vi "Begin.vi"(8 "error in (no error)":errorcluster, 11 "Elevator Concrete in":refnum<class "Elevator Concrete.lvclass">) -> (0 "error out":errorcluster, 3 "Elevator Concrete out":refnum<class "Elevator Concrete.lvclass">)   [LabVIEW 2018, in "Elevator.lvlib" / "Elevator Concrete.lvclass"]
uses:
  Elevator Concrete.lvclass
  C:/Users/Public/Documents/2019DeepSpace/Classes/Elevator/Elevator.lvclass
  <vilib>/Rock Robotics/WPI/ThirdParty/Phoenix-LabVIEW/Motor Controller/Controls/CTRE_Phoenix_MotorControl_EnhancedMotorControllerConfigurables.ctl
  <vilib>/Rock Robotics/WPI/ThirdParty/Phoenix-LabVIEW/Motor Controller/Controls/CTRE_Phoenix_MotorControl_BaseConfigurables.ctl
  <vilib>/Rock Robotics/WPI/ThirdParty/Phoenix-LabVIEW/Motor Controller/Controls/CTRE_Phoenix_MotorControl_VelocityMeasurementPeriod.ctl
  <vilib>/Rock Robotics/WPI/ThirdParty/Phoenix-LabVIEW/Motor Controller/Controls/CTRE_Phoenix_MotorControl_SlotStructure.ctl
  <vilib>/Rock Robotics/WPI/ThirdParty/Phoenix-LabVIEW/Motor Controller/Controls/CTRE_Phoenix_MotorControl_FilterStruct.ctl
  <vilib>/Rock Robotics/WPI/ThirdParty/Phoenix-LabVIEW/Motor Controller/Controls/CTRE_Phoenix_MotorControl_RemoteSourceType.ctl
  <vilib>/Rock Robotics/WPI/ThirdParty/Phoenix-LabVIEW/Controls/CTRE_Phoenix_CustomParamConfiguration.ctl
  <vilib>/Rock Robotics/WPI/ThirdParty/Phoenix-LabVIEW/Motor Controller/Controls/CTRE_Phoenix_MotorControl_FeedbackDevice.ctl
  <vilib>/Rock Robotics/WPI/ThirdParty/Phoenix-LabVIEW/Motor Controller/Controls/CTRE_Phoenix_MotorControl_SensorTermFeedbackDevice_Enhanced.ctl
  <vilib>/Rock Robotics/WPI/ThirdParty/Phoenix-LabVIEW/Motor Controller/Controls/CTRE_Phoenix_MotorControl_LimitSwitchNormal.ctl
  <vilib>/Rock Robotics/WPI/ThirdParty/Phoenix-LabVIEW/Motor Controller/Controls/CTRE_Phoenix_MotorControl_LimitSwitchSource_Local.ctl
  Elevator Concrete.lvclass/Elevator Concrete.ctl
  <vilib>/Rock Robotics/WPI/ThirdParty/Phoenix-LabVIEW/Motor Controller/Get/CTRE_Phoenix_MotorController_GetPulseWidthAll.vi
  Elevator.lvclass
panel:
  out "Pulse Width Rise-to-Rise Time (us)":i32
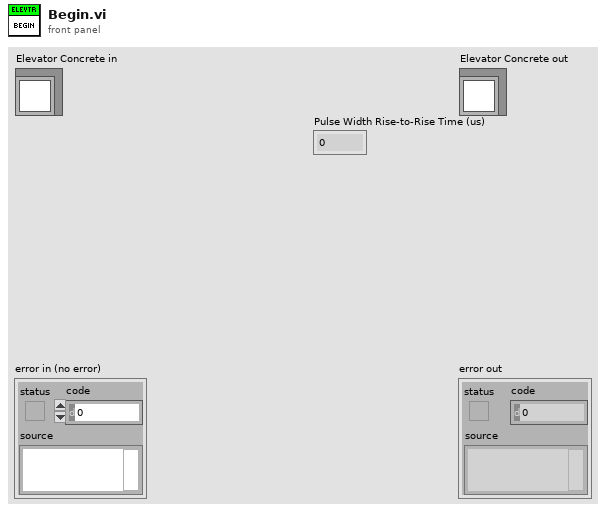
[diagram p1: front panel]
types:
  T1 = typedef "CTRE_Phoenix_MotorControl_EnhancedMotorControllerConfigurables.ctl" = cluster{"Base Configurables":T2, "primaryPID":cluster{"selectedFeedbackCoefficient":dbl, "selectedFeedbackSensor":T8}, "auxiliaryPID":cluster{"selectedFeedbackCoefficient":dbl, "selectedFeedbackSensor":T8}, "sum0Term":T9, "sum1Term":T9, "diff0Term":T9, "diff1Term":T9, "forwardLimitSwitchNormal":T10, "reverseLimitSwitchNormal":T10, "forwardLimitSwitchDeviceID":i32, "reverseLimitSwitchDeviceID":i32, "forwardLimitSwitchSource":T11, "reverseLimitSwitchSource":T11, "peakCurrentLimit":i32, "peakCurrentDuration":i32, "continuousCurrentLimit":i32}
  T2 = typedef "CTRE_Phoenix_MotorControl_BaseConfigurables.ctl" = cluster{"openLoopRamp":dbl, "closedLoopRamp":dbl, "peakOutputForward":dbl, "peakOutputReverse":dbl, "nominalOutputForward":dbl, "nominalOutputReverse":dbl, "neutralDeadband":dbl, "voltageCompSaturation":dbl, "voltageMeasurementFilter":i32, "velocityMeasurementPeriod":T3, "velocityMeasurementWindow":i32, "forwardSoftLimitThreshold":i32, "reverseSoftLimitThreshold":i32, "forwardSoftLimitEnable":bool, "reverseSoftLimitEnable":bool, "slot0":T4, "slot1":T4, "slot2":T4, "slot3":T4, "auxPIDPolarity":bool, "remoteFilter0":T5, "remoteFilter1":T5, "motionCruiseVelocity":i32, "motionAcceleration":i32, "motionProfileTrajectoryPeriod":i32, "feedbackNotContinuous":bool, "remoteSensorClosedLoopDisableNeutralOnLOS":bool, "clearPositionOnLimitF":bool, "clearPositionOnLimitR":bool, "clearPositionOnQuadIdx":bool, "limitSwitchDisableNeutralOnLOS":bool, "softLimitDisableNeutralOnLOS":bool, "pulseWidthPeriod_EdgesPerRot":i32, "pulseWidthPeriod_FilterWindowSz":i32, "customParam":T7, "trajectoryInterpolationEnable":bool}
  T3 = typedef "CTRE_Phoenix_MotorControl_VelocityMeasurementPeriod.ctl" = u16
  T4 = typedef "CTRE_Phoenix_MotorControl_SlotStructure.ctl" = cluster{"P":dbl, "I":dbl, "D":dbl, "F":dbl, "integralZone":dbl, "allowableClosedLoopError":i32, "maxIntegralAccumulator":dbl, "closedLoopPeakOutput":dbl, "closedLoopPeriod":i32}
  T5 = typedef "CTRE_Phoenix_MotorControl_FilterStruct.ctl" = cluster{"remoteSensorDeviceID":u8, "remoteSensorSource":T6}
  T6 = typedef "CTRE_Phoenix_MotorControl_RemoteSourceType.ctl" = enum16{"Off", "Talon SRX Selected Sensor", "Pigeon IMU Yaw", "Pigeon IMU Pitch", "Pigeon IMU Roll", "CANifier Quadrature", "CANifier PWM Input 0", "CANifier PWM Input 1", "CANifier PWM Input 2", "CANifier PWM Input 3", "Gadgeteer Pigeon Yaw", "Gadgeteer Pigeon Pitch", "Gadgeteer Pigeon Roll"}
  T7 = typedef "CTRE_Phoenix_CustomParamConfiguration.ctl" = cluster{"customParam0":i32, "customParam1":i32}
  T8 = typedef "CTRE_Phoenix_MotorControl_FeedbackDevice.ctl" = i8
  T9 = typedef "CTRE_Phoenix_MotorControl_SensorTermFeedbackDevice_Enhanced.ctl" = i8
  T10 = typedef "CTRE_Phoenix_MotorControl_LimitSwitchNormal.ctl" = enum16{"Normally Open", "Normally Closed", "Disabled"}
  T11 = typedef "CTRE_Phoenix_MotorControl_LimitSwitchSource_Local.ctl" = enum16{"Feedback Connector", "Remote Talon SRX", "Remote CANifier", "Deactivated"}
  T12 = typedef "Elevator.lvlib/Elevator.lvclass/Elevator IDs.ctl" = cluster{"Wrist":u8, "Left Master":u8, "Left Slave":u8, "Right Master":u8, "Right Slave":u8, "Vacumm Pump 1":u8, "Vacumm Pump 2":u8}
  T13 = typedef "Elevator.lvlib/Elevator.lvclass/Elevator Constants.ctl" = cluster{"Arm Motion Magic Max Velocity":u32, "Arm Motion Magic Max Acceleration":u32, "Wrist Motion Magic Max Velocity":u32, "Wrist Motion Magic Max Acceleration":u32, "Arm Gear Ratio":dbl, "Wrist Gear Ratio":dbl, "Arm Encoder ABS Value":i32, "Wrist Encoder ABS Value":i32}
  T14 = typedef "WPI_MotorControlDeviceRef.ctl" = cluster{"DeviceStatus":errorcluster, "Type":T15, "PWM":cluster{"PWM Channel":T16, "DeadBand":T17}, "CAN":cluster{"Device Number":u8, "SetOutput VI Ref":variant, "GetOutput VI Ref":variant, "Enable VI Ref":variant, "Disable VI Ref":variant, "Data":variant}, "Invert":bool, "DIO PWM":cluster{"PWM \"Enable\" Channel":T16, "DIOChannel":T18, "PWM Rate":dbl}}
  T15 = typedef "WPI_MotorControlType.ctl" = enum16{"PWM", "CAN", "DIO PWM"}
  T16 = typedef "FPGA_DIOPWMChannel.ctl" = enum8{"PWM 0", "PWM 1", "PWM 2", "PWM 3", "PWM 4", "PWM 5", "PWM 6", "PWM 7", "PWM 8", "PWM 9", "PWM MXP 0", "PWM MXP 1", "PWM MXP 2", "PWM MXP 3", "PWM MXP 4", "PWM MXP 5", "PWM MXP 6", "PWM MXP 7", "PWM MXP 8", "PWM MXP 9", "Invalid"}
  T17 = typedef "WPI_PWMDeadband.ctl" = cluster{"Name":string, "maxPositivePwm":i32, "minPositivePwm":i32, "centerPwm":i32, "maxNegativePwm":i32, "minNegativePwm":i32, "angularRange":u16}
  T18 = typedef "FPGA_DIOChannel.ctl" = enum8{"DIO 0", "DIO 1", "DIO 2", "DIO 3", "DIO 4", "DIO 5", "DIO 6", "DIO 7", "DIO 8", "DIO 9", "DIO MXP 0", "DIO MXP 1", "DIO MXP 2", "DIO MXP 3", "DIO MXP 4", "DIO MXP 5", "DIO MXP 6", "DIO MXP 7", "DIO MXP 8", "DIO MXP 9", "DIO MXP 10", "DIO MXP 11", "DIO MXP 12", "DIO MXP 13", "DIO MXP 14", "DIO MXP 15", "SPI Port CS1", "SPI Port CS2", "SPI Port CS3", "SPI Port MISO", "SPI Port MOSI", "Invalid"}
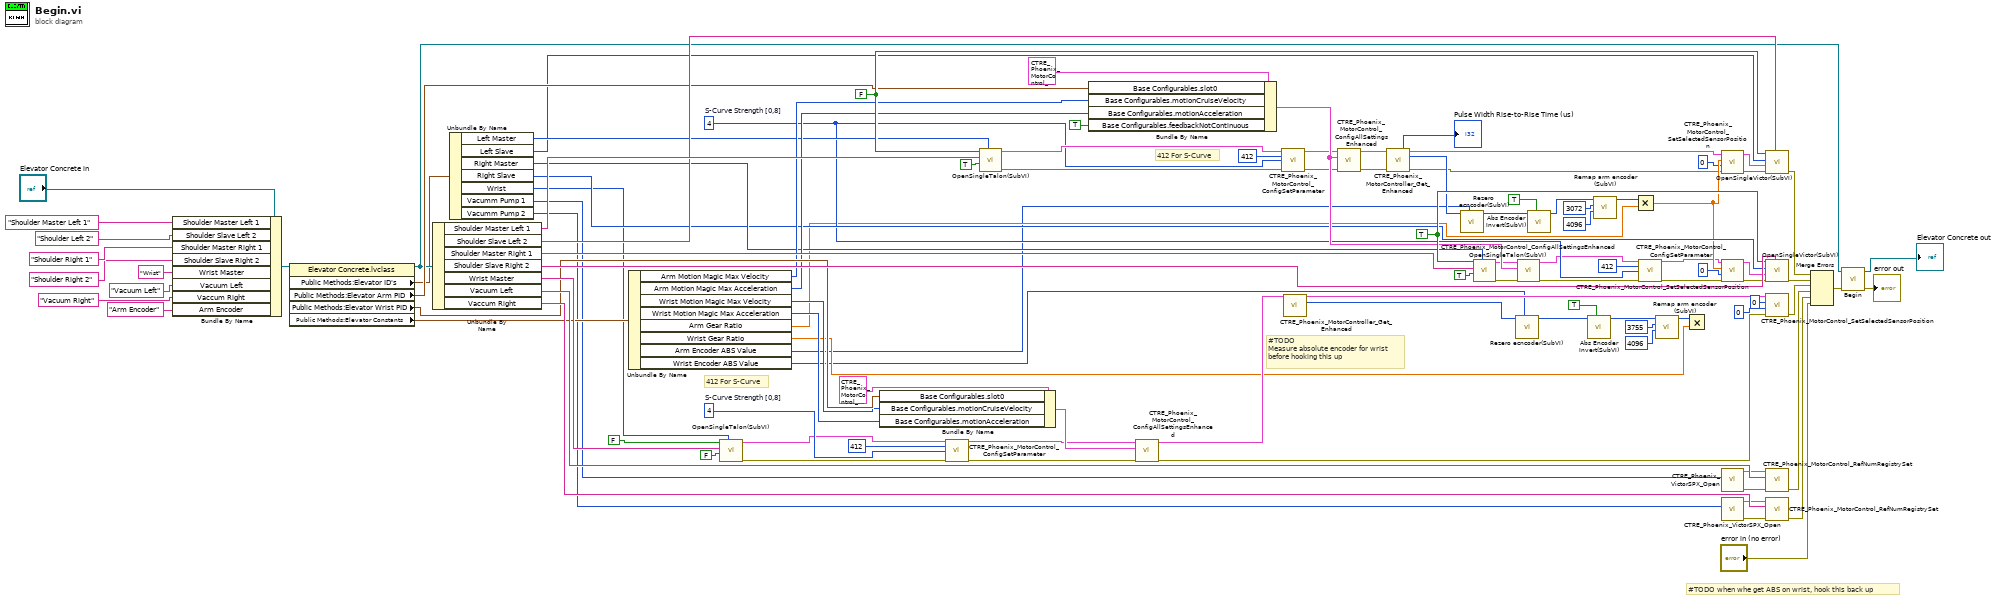
[diagram p0: block diagram]
diagram:
  w25 = 4  # S-Curve Strength [0,8]
  w30 = 4  # S-Curve Strength [0,8]
  w70 = FALSE ("invert")
  w86 = TRUE ("Invert?")
  # "#TODO when whe get ABS on wrist, hook this back up"
  # "#TODO \nMeasure absolute encoder for wrist\nbefore hooking this up"
  # "412 For S-Curve"
  # "412 For S-Curve"
  n1 = Bundle By Name(cluster="Elevator Concrete in", "Shoulder Master Left 1"="Shoulder Master Left 1" ("Shoulder Slave Left 1"), "Shoulder Slave Left 2"="Shoulder Left 2", "Shoulder Master Right 1"="Shoulder Right 1", "Shoulder Slave Right 2"="Shoulder Right 2", "Wrist Master"="Wrist", "Vacuum Left"="Vacuum Left", "Vaccum Right"="Vacuum Right", "Arm Encoder"="Arm Encoder") -> (w65:refnum<class "Elevator Concrete.lvclass">)
  n2 = property class="Elevator Concrete.lvclass"(reference=w65) -> (reference out=w62:refnum<class "Elevator Concrete.lvclass">, "Public Methods:Elevator ID's"=w56:T12, "Public Methods:Elevator Arm PID"=w64:T4, "Public Methods:Elevator Wrist PID"=w63:T4, "Public Methods:Elevator Constants"=w61:T13)  [unwired: 1 in, 1 out]
  n3 = Unbundle By Name(w62) -> ("Shoulder Master Left 1"=w105:string, "Shoulder Slave Left 2"=w104:string, "Shoulder Master Right 1"=w103:string, "Shoulder Slave Right 2"=w102:string, "Wrist Master"=w101:string, "Vacuum Left"=w100:string, "Vaccum Right"=w99:string)
  n4 = Unbundle By Name(w56) -> ("Left Master"=w53:u8, "Left Slave"=w52:u8, "Right Master"=w51:u8, "Right Slave"=w50:u8, "Wrist"=w49:u8, "Vacumm Pump 1"=w54:u8, "Vacumm Pump 2"=w55:u8)
  n5 = Unbundle By Name(w61) -> ("Arm Motion Magic Max Velocity"=w60:u32, "Arm Motion Magic Max Acceleration"=w59:u32, "Wrist Motion Magic Max Velocity"=w58:u32, "Wrist Motion Magic Max Acceleration"=w57:u32, "Arm Gear Ratio"=w5:dbl, "Wrist Gear Ratio"=w4:dbl, "Arm Encoder ABS Value"=w3:i32, "Wrist Encoder ABS Value"=w2:i32)
  n6 = call "OpenSingleTalon(SubVI).vi"("can_id"=w49, "sensor_phase"=FALSE, "refnum name"=w101, "invert"=FALSE) -> ("error out"=w22:errorcluster, "PhoenixMotorControlDevRef"=w24:T14)  [unwired: 6 in]
  n7 = Bundle By Name(cluster=T1 {"Base Configurables"={"openLoopRamp"=0.0, "closedLoopRamp"=0.0, "peakOutputForward"=1.0, "peakOutputReverse"=-1.0, "nominalOutputForward"=0.0, "nominalOutputReverse"=0.0, "neutralDeadband"=0.04, "voltageCompSaturation"=0.0, "voltageMeasurementFilter"=32, "velocityMeasurementPeriod"=100, "velocityMeasurementWindow"=64, "forwardSoftLimitThreshold"=0, "reverseSoftLimitThreshold"=0, "forwardSoftLimitEnable"=FALSE, "reverseSoftLimitEnable"=FALSE, "slot0"={"P"=0.0, "I"=0.0, "D"=0.0, "F"=0.0, "integralZone"=0.0, "allowableClosedLoopError"=0, "maxIntegralAccumulator"=0.0, "closedLoopPeakOutput"=1.0, "closedLoopPeriod"=1}, "slot1"={"P"=0.0, "I"=0.0, "D"=0.0, "F"=0.0, "integralZone"=0.0, "allowableClosedLoopError"=0, "maxIntegralAccumulator"=0.0, "closedLoopPeakOutput"=1.0, "closedLoopPeriod"=1}, "slot2"={"P"=0.0, "I"=0.0, "D"=0.0, "F"=0.0, "integralZone"=0.0, "allowableClosedLoopError"=0, "maxIntegralAccumulator"=0.0, "closedLoopPeakOutput"=1.0, "closedLoopPeriod"=1}, "slot3"={"P"=0.0, "I"=0.0, "D"=0.0, "F"=0.0, "integralZone"=0.0, "allowableClosedLoopError"=0, "maxIntegralAccumulator"=0.0, "closedLoopPeakOutput"=1.0, "closedLoopPeriod"=1}, "auxPIDPolarity"=FALSE, "remoteFilter0"={"remoteSensorDeviceID"=0, "remoteSensorSource"=enum."Off"}, "remoteFilter1"={"remoteSensorDeviceID"=0, "remoteSensorSource"=enum."Off"}, "motionCruiseVelocity"=0, "motionAcceleration"=0, "motionProfileTrajectoryPeriod"=0, "feedbackNotContinuous"=FALSE, "remoteSensorClosedLoopDisableNeutralOnLOS"=FALSE, "clearPositionOnLimitF"=FALSE, "clearPositionOnLimitR"=FALSE, "clearPositionOnQuadIdx"=FALSE, "limitSwitchDisableNeutralOnLOS"=FALSE, "softLimitDisableNeutralOnLOS"=FALSE, "pulseWidthPeriod_EdgesPerRot"=1, "pulseWidthPeriod_FilterWindowSz"=1, "customParam"={"customParam0"=0, "customParam1"=0}, "trajectoryInterpolationEnable"=TRUE}, "primaryPID"={"selectedFeedbackCoefficient"=1.0, "selectedFeedbackSensor"=0}, "auxiliaryPID"={"selectedFeedbackCoefficient"=1.0, "selectedFeedbackSensor"=0}, "sum0Term"=0, "sum1Term"=0, "diff0Term"=0, "diff1Term"=0, "forwardLimitSwitchNormal"=enum."Normally Open", "reverseLimitSwitchNormal"=enum."Normally Open", "forwardLimitSwitchDeviceID"=0, "reverseLimitSwitchDeviceID"=0, "forwardLimitSwitchSource"=enum."Feedback Connector", "reverseLimitSwitchSource"=enum."Feedback Connector", "peakCurrentLimit"=1, "peakCurrentDuration"=1, "continuousCurrentLimit"=1} ("Enhanced Motor Controller Configurables"), "Base Configurables.slot0"=w63, "Base Configurables.motionCruiseVelocity"=w58, "Base Configurables.motionAcceleration"=w57) -> (w73:T1)
  n8 = call <vilib>:"CTRE_Phoenix_MotorControl_ConfigSetParameter.vi"("PhoenixMotorControlDevRef"=w24, "Parameter"=u32 412 ("subValue"), "value"=w25, "error in (no error)"=w22) -> ("PhoenixMotorControlDevRef"=w23:T14, "error out"=w21:errorcluster)  [unwired: 10 in]
  n9 = call "OpenSingleTalon(SubVI).vi"("can_id"=w53, "sensor_phase"=TRUE, "refnum name"=w105, "invert"=w70) -> ("error out"=w32:errorcluster, "PhoenixMotorControlDevRef"=w34:T14)  [unwired: 6 in]
  n10 = Bundle By Name(cluster=T1 {"Base Configurables"={"openLoopRamp"=0.0, "closedLoopRamp"=0.0, "peakOutputForward"=1.0, "peakOutputReverse"=-1.0, "nominalOutputForward"=0.0, "nominalOutputReverse"=0.0, "neutralDeadband"=0.04, "voltageCompSaturation"=0.0, "voltageMeasurementFilter"=32, "velocityMeasurementPeriod"=100, "velocityMeasurementWindow"=64, "forwardSoftLimitThreshold"=0, "reverseSoftLimitThreshold"=0, "forwardSoftLimitEnable"=FALSE, "reverseSoftLimitEnable"=FALSE, "slot0"={"P"=0.0, "I"=0.0, "D"=0.0, "F"=0.0, "integralZone"=0.0, "allowableClosedLoopError"=0, "maxIntegralAccumulator"=0.0, "closedLoopPeakOutput"=1.0, "closedLoopPeriod"=1}, "slot1"={"P"=0.0, "I"=0.0, "D"=0.0, "F"=0.0, "integralZone"=0.0, "allowableClosedLoopError"=0, "maxIntegralAccumulator"=0.0, "closedLoopPeakOutput"=1.0, "closedLoopPeriod"=1}, "slot2"={"P"=0.0, "I"=0.0, "D"=0.0, "F"=0.0, "integralZone"=0.0, "allowableClosedLoopError"=0, "maxIntegralAccumulator"=0.0, "closedLoopPeakOutput"=1.0, "closedLoopPeriod"=1}, "slot3"={"P"=0.0, "I"=0.0, "D"=0.0, "F"=0.0, "integralZone"=0.0, "allowableClosedLoopError"=0, "maxIntegralAccumulator"=0.0, "closedLoopPeakOutput"=1.0, "closedLoopPeriod"=1}, "auxPIDPolarity"=FALSE, "remoteFilter0"={"remoteSensorDeviceID"=0, "remoteSensorSource"=enum."Off"}, "remoteFilter1"={"remoteSensorDeviceID"=0, "remoteSensorSource"=enum."Off"}, "motionCruiseVelocity"=0, "motionAcceleration"=0, "motionProfileTrajectoryPeriod"=0, "feedbackNotContinuous"=FALSE, "remoteSensorClosedLoopDisableNeutralOnLOS"=FALSE, "clearPositionOnLimitF"=FALSE, "clearPositionOnLimitR"=FALSE, "clearPositionOnQuadIdx"=FALSE, "limitSwitchDisableNeutralOnLOS"=FALSE, "softLimitDisableNeutralOnLOS"=FALSE, "pulseWidthPeriod_EdgesPerRot"=1, "pulseWidthPeriod_FilterWindowSz"=1, "customParam"={"customParam0"=0, "customParam1"=0}, "trajectoryInterpolationEnable"=TRUE}, "primaryPID"={"selectedFeedbackCoefficient"=1.0, "selectedFeedbackSensor"=0}, "auxiliaryPID"={"selectedFeedbackCoefficient"=1.0, "selectedFeedbackSensor"=0}, "sum0Term"=0, "sum1Term"=0, "diff0Term"=0, "diff1Term"=0, "forwardLimitSwitchNormal"=enum."Normally Open", "reverseLimitSwitchNormal"=enum."Normally Open", "forwardLimitSwitchDeviceID"=0, "reverseLimitSwitchDeviceID"=0, "forwardLimitSwitchSource"=enum."Feedback Connector", "reverseLimitSwitchSource"=enum."Feedback Connector", "peakCurrentLimit"=1, "peakCurrentDuration"=1, "continuousCurrentLimit"=1} ("Enhanced Motor Controller Configurables"), "Base Configurables.slot0"=w64, "Base Configurables.motionCruiseVelocity"=w60, "Base Configurables.motionAcceleration"=w59, "Base Configurables.feedbackNotContinuous"=TRUE) -> (w84:T1)
  n11 = call <vilib>:"CTRE_Phoenix_MotorControl_ConfigAllSettingsEnhanced.vi"("error in (no error)"=w21, "Enhanced Motor Controller Configurables"=w73, "PhoenixMotorControlDevRef"=w23) -> ("error out"=w74:errorcluster, "PhoenixMotorControlDevRef"=w17:T14)  [unwired: 7 in]
  n12 = call <vilib>:"CTRE_Phoenix_MotorControl_ConfigSetParameter.vi"("PhoenixMotorControlDevRef"=w34, "Parameter"=u32 412 ("subValue"), "value"=w30, "error in (no error)"=w32) -> ("PhoenixMotorControlDevRef"=w33:T14, "error out"=w31:errorcluster)  [unwired: 10 in]
  n13 = call-poly <vilib>:"CTRE_Phoenix_MotorController_Get_Enhanced.vi"("PhoenixMotorControlDevRef"=w17) -> ("PhoenixMotorControlDevRef"=w16:T14, "Pulse Width Position"=w15:i32)  [unwired: 9 in, 4 out]
  n14 = call <vilib>:"CTRE_Phoenix_MotorControl_ConfigAllSettingsEnhanced.vi"("error in (no error)"=w31, "Enhanced Motor Controller Configurables"=w84, "PhoenixMotorControlDevRef"=w33) -> ("error out"=w36:errorcluster, "PhoenixMotorControlDevRef"=w38:T14)  [unwired: 7 in]
  n15 = call-poly <vilib>:"CTRE_Phoenix_MotorController_Get_Enhanced.vi"("PhoenixMotorControlDevRef"=w38, "error in"=w36) -> ("Pulse Width Rise-to-Rise Time (us)"=→"Pulse Width Rise-to-Rise Time (us)":i32, "PhoenixMotorControlDevRef"=w37:T14, "Pulse Width Position"=w48:i32, "error out"=w35:errorcluster)  [unwired: 8 in, 2 out]
  n16 = call "Rezero ecncoder(SubVI).vi"("Zero"=w3, "Encoder"=w48) -> ("Rezeroed Encoder"=w39:i32)  [unwired: 9 in]
  n17 = call "OpenSingleTalon(SubVI).vi"("can_id"=w51, "sensor_phase"=TRUE, "refnum name"=w103, "invert"=w86) -> ("error out"=w87:errorcluster, "PhoenixMotorControlDevRef"=w66:T14)  [unwired: 6 in]
  n18 = call "Rezero ecncoder(SubVI).vi"("Zero"=w2, "Encoder"=w15) -> ("Rezeroed Encoder"=w20:i32)  [unwired: 9 in]
  n19 = call <vilib>:"CTRE_Phoenix_MotorControl_ConfigAllSettingsEnhanced.vi"("error in (no error)"=w87, "Enhanced Motor Controller Configurables"=w84, "PhoenixMotorControlDevRef"=w66) -> ("error out"=w27:errorcluster, "PhoenixMotorControlDevRef"=w29:T14)  [unwired: 7 in]
  n20 = call "Abs Encoder Invert(SubVI).vi"("Sensor Phase"=TRUE, "encoder"=w39) -> ("encoder reversed"=w41:i32)  [unwired: 9 in]
  n21 = call "Abs Encoder Invert(SubVI).vi"("Sensor Phase"=TRUE, "encoder"=w20) -> ("encoder reversed"=w11:i32)  [unwired: 9 in]
  n22 = call "Remap arm encoder (SubVI).vi"("encoder ticks per revolution"=4096, "crossover to negative"=3072, "Value"=w41) -> ("Mapped"=w44:i32)  [unwired: 8 in]
  n23 = Multiply(x=w44, y=w5) -> (x*y=w45:dbl)
  n24 = call <vilib>:"CTRE_Phoenix_MotorControl_ConfigSetParameter.vi"("PhoenixMotorControlDevRef"=w29, "Parameter"=u32 412 ("subValue"), "value"=w30, "error in (no error)"=w27) -> ("PhoenixMotorControlDevRef"=w28:T14, "error out"=w26:errorcluster)  [unwired: 10 in]
  n25 = call "Remap arm encoder (SubVI).vi"("encoder ticks per revolution"=4096, "crossover to negative"=3755, "Value"=w11) -> ("Mapped"=w10:i32)  [unwired: 8 in]
  n26 = Multiply(x=w10, y=w4) -> ()  [unwired: 1 out]
  n27 = call <vilib>:"CTRE_Phoenix_MotorControl_SetSelectedSensorPosition.vi"("error in (no error)"=w35, "pidLoopIdx"=u32 0, "New Sensor Position"=w45, "PhoenixMotorControlDevRef"=w37) -> ("error out"=w107:errorcluster, "PhoenixMotorControlDevRef"=w106:T14)  [unwired: 6 in]
  n28 = call <vilib>:"CTRE_Phoenix_MotorControl_SetSelectedSensorPosition.vi"("error in (no error)"=w26, "pidLoopIdx"=u32 0, "New Sensor Position"=w45, "PhoenixMotorControlDevRef"=w28) -> ("error out"=w89:errorcluster, "PhoenixMotorControlDevRef"=w88:T14)  [unwired: 6 in]
  n29 = call <vilib>:"CTRE_Phoenix_VictorSPX_Open.vi"("Device Number"=w54) -> ("error out"=w78:errorcluster, "CAN Talon SRX Ref"=w77:T14)  [unwired: 9 in]
  n30 = call <vilib>:"CTRE_Phoenix_VictorSPX_Open.vi"("Device Number"=w55) -> ("error out"=w81:errorcluster, "CAN Talon SRX Ref"=w80:T14)  [unwired: 9 in]
  n31 = call "OpenSingleVictor(SubVI).vi"("refnum name"=w104, "error in (no error)"=w107, "Master Controller to Follow"=w106, "Device Number"=w52, "Invert?"=w70) -> ("error out"=w108:errorcluster)  [unwired: 5 in, 1 out]
  n32 = call "OpenSingleVictor(SubVI).vi"("refnum name"=w102, "error in (no error)"=w89, "Master Controller to Follow"=w88, "Device Number"=w50, "Invert?"=w86) -> ("error out"=w90:errorcluster)  [unwired: 5 in, 1 out]
  n33 = call <vilib>:"CTRE_Phoenix_MotorControl_SetSelectedSensorPosition.vi"("error in (no error)"=w74, "pidLoopIdx"=0 ("New Sensor Position"), "New Sensor Position"=0, "PhoenixMotorControlDevRef"=w16) -> ("error out"=w71:errorcluster)  [unwired: 6 in, 1 out]
  n34 = call <vilib>:"CTRE_Phoenix_MotorControl_RefNumRegistrySet.vi"("error in (no error)"=w78, "refnum name"=w100, "PhoenixMotorControlDevRef"=w77) -> ("error out"=w79:errorcluster)  [unwired: 7 in, 1 out]
  n35 = call <vilib>:"CTRE_Phoenix_MotorControl_RefNumRegistrySet.vi"("error in (no error)"=w81, "refnum name"=w99, "PhoenixMotorControlDevRef"=w80) -> ("error out"=w82:errorcluster)  [unwired: 7 in, 1 out]
  n36 = Merge Errors(w108, w90, w71, w79, w82, "error in (no error)") -> (w109:errorcluster)
  n37 = call-parent "Begin.vi"("error in (no error)"=w109, "Elevator in"=w62) -> ("error out"=→"error out":errorcluster, "Elevator out"=→"Elevator Concrete out":refnum<class "Elevator Concrete.lvclass">)  [unwired: 8 in]
